vi "DELETE ME SLM.vi"() -> ()   [LabVIEW 2012]
panel:
  out "initialized array":dbl[][](array[numeric])
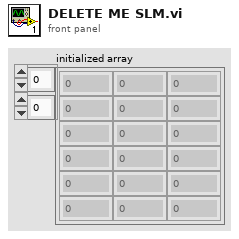
[diagram p1: front panel]
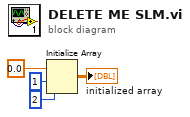
[diagram p0: block diagram]
diagram:
  n1 = Initialize Array(0.0 ("element"), 1 ("dimension size"), 2 ("dimension size")) -> (→"initialized array":dbl[][])
